vi "read.issue_ids.from.volume.vi"(8 "error in":errorcluster, 11 "file (use dialog)":path) -> (0 "error out":errorcluster, 3 "issue_ids":i32[](array[numeric]))   [LabVIEW 2024]
uses:
  <vilib>/addons/_JKI.lib/Serialization/JSON/JKI JSON Serialization.lvlib
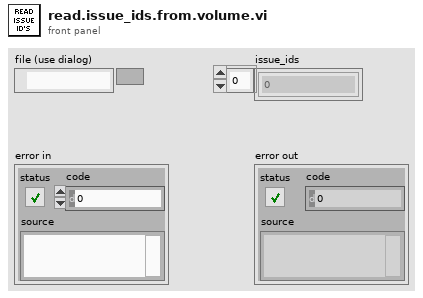
[diagram p1: front panel]
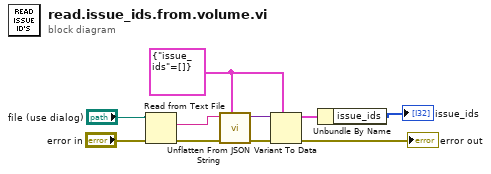
[diagram p0: block diagram]
diagram:
  w4 = cluster{"issue_ids":i32[]} {"issue_ids"=[]}
  n1 = Read from Text File(file (use dialog)="file (use dialog)", error in="error in") -> (text=w8:string, error out=w7:errorcluster)  [unwired: 2 in, 2 out]
  n2 = call <vilib>:"Unflatten From JSON String.vi"("Type and Defaults"=w4, "error in (no error)"=w7, "JSON String"=w8) -> ("error out"=w6:errorcluster, "Variant"=w5:variant)  [unwired: 7 in]
  n3 = Variant To Data(error in=w6, type=w4, Variant=w5) -> (data=w3:cluster{"issue_ids":i32[]}, error out=→"error out":errorcluster)
  n4 = Unbundle By Name(w3) -> ("issue_ids"=→"issue_ids":i32[])
